vi "Update Chronometer Display.vi"(8 "error in (no error)":errorcluster, 11 "Chronometer in":refnum<class "Chronometer.lvclass">) -> (0 "error out":errorcluster, 3 "Chronometer out":refnum<class "Chronometer.lvclass">)   [LabVIEW 2023, in "Chronometer.lvlib" / "Chronometer.lvclass"]
uses:
  Library/Chronometer.lvclass
  Library/Chronometer.lvclass/Chronometer.ctl
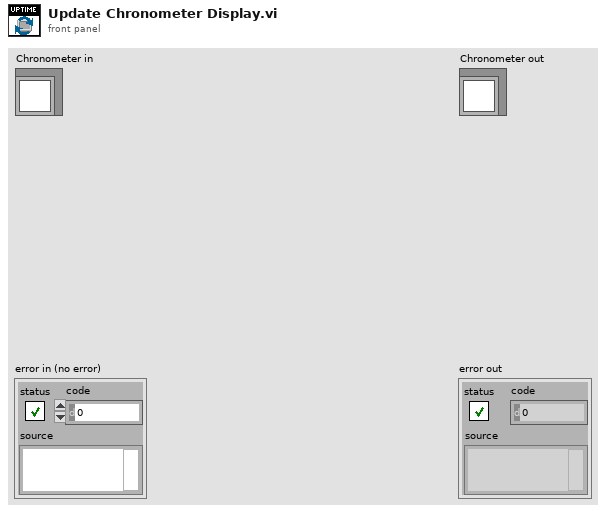
[diagram p1: front panel]
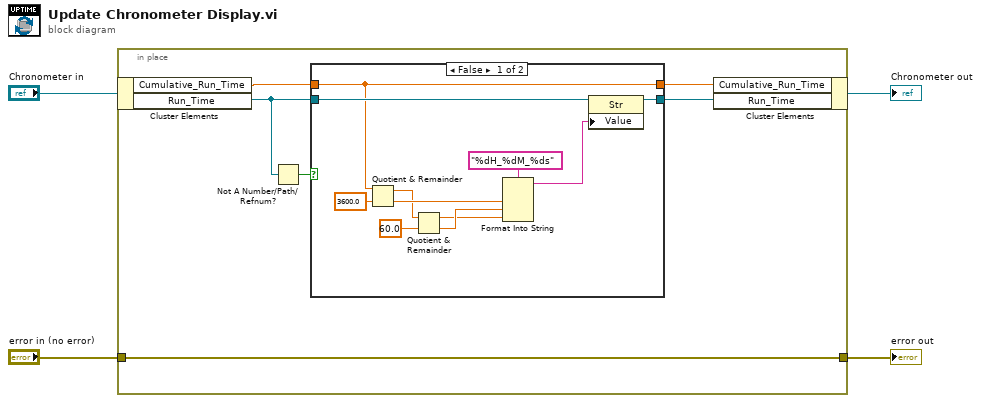
[diagram p0: block diagram]
diagram:
  n1 = in-place {
    in-place-border: "error in (no error)" -> [w10]
    in-place-border: [w10] -> w1
    n2 = in-place-cluster #1("Chronometer in") -> ("Cumulative_Run_Time"=w9:dbl, "Run_Time"=w7:refnum<vi>)
    n3 = Not A Number/Path/Refnum?(number/path/refnum=w7) -> (NaN/Path/Refnum?=w6:bool)
    n4 = case shown="False" w6 {
      tunnel: w9 -> [w11 w22]
      tunnel: [w14 w23] -> w8
      tunnel: w7 -> [w12 w23]
      tunnel: [w11 w22] -> w5
      frame False {
        n5 = Quotient & Remainder(x=w11, y=3600.0) -> (x-y*floor(x/y)=w18:dbl, floor(x/y)=w19:dbl)
        n6 = Quotient & Remainder(x=w18, y=60.0) -> (x-y*floor(x/y)=w15:dbl, floor(x/y)=w16:dbl)
        n7 = Format Into String(format string="%dH_%dM_%ds", w19, w16, w15) -> (resulting string=w13:string)  [unwired: 2 in, 1 out]
        n8 = property class="Str"(reference=w12, "Value"=w13) -> (reference out=w14:refnum<vi>)  [unwired: 1 in, 1 out]
      }
      frame True {
      }
    }
    n9 = in-place-cluster #1("Cumulative_Run_Time"=w5, "Run_Time"=w8) -> (→"Chronometer out":refnum<class "Chronometer.lvclass">)
  }
  "error out" <- w1
